vi "rx streamer num channels.vi"(8 "error in (no error)":errorcluster, 10 "num_channels_out":u64, 11 "h":u64) -> (0 "error out":errorcluster, 2 "num_channels_out out":u64, 3 "function return":u32(ring))   [LabVIEW 2023, in "uhd.lvlib"]
doc: "UHD_API uhd_error uhd_rx_streamer_num_channels(\n uhd_rx_streamer_handle h, size_t* num_channels_out);"
uses:
  <userlib>/uhd/uhd.lvlib
  <userlib>/uhd/uhd.dll
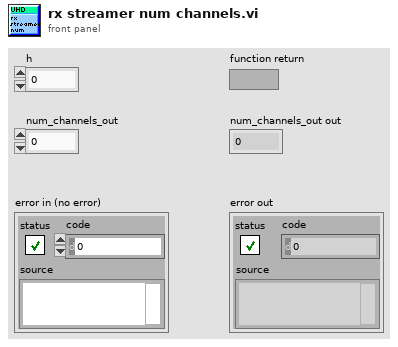
[diagram p1: front panel]
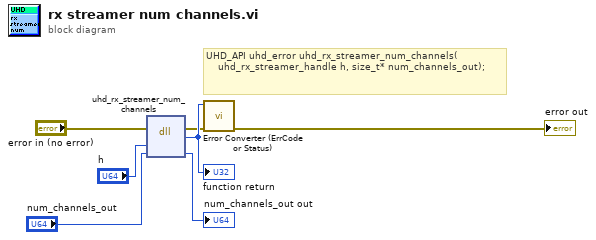
[diagram p0: block diagram]
diagram:
  # "UHD_API uhd_error uhd_rx_streamer_num_channels(\n    uhd_rx_streamer_handle h, size_t* num_channels_out);"
  n1 = dll-call lib="C:/Program Files/National Instruments/LabVIEW 2023/user.lib/uhd/uhd.*" fn="uhd_rx_streamer_num_channels"(error in="error in (no error)", "h"="h", "num_channels_out"="num_channels_out") -> (error out=w2:errorcluster, w7:u32, "num_channels_out"=→"num_channels_out out":u64)  [unwired: 3 in, 1 out]
  "function return" <- w7
  n2 = call <userlib>:"Error Converter (ErrCode or Status).vi"("error in (no error)"=w2, "error code"=w7) -> ("error out"=→"error out":errorcluster)  [unwired: 9 in]
